vi "Auto_Drive (2).vi"(10 "Target":dbl=40.0 format="%#_13g", 11 "Drive Effort":dbl=0.1) -> ()   [LabVIEW 2016]
uses:
  <vilib>/Rock Robotics/WPI/SafetyOutput/WPI_SafetyOutputConfigMenu.ctl
  Global 2.vi
panel:
  in  "kI":dbl=1.6 format="%#_13g"
  in  "kP":dbl=0.35 format="%#_13g"
  in  "kD":dbl=1.6 format="%#_13g"
  in  "Scaling Factor":dbl=16.0 format="%#_13g"
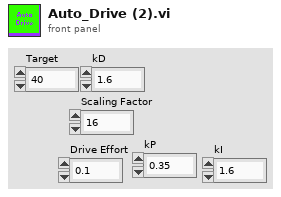
[diagram p1: front panel]
types:
  T1 = typedef "WPI_SafetyOutputConfigMenu.ctl" = enum16{"Enable", "Disable"}
  T2 = typedef "WPI_MotorControlDeviceRef.ctl" = cluster{"DeviceStatus":errorcluster, "Type":T3, "PWM":cluster{"PWM Channel":T4, "DeadBand":T5}, "CAN":cluster{"Device Number":u8, "SetOutput VI Ref":variant, "GetOutput VI Ref":variant, "Enable VI Ref":variant, "Disable VI Ref":variant, "Data":variant}, "Invert":bool}
  T3 = typedef "WPI_MotorControlType.ctl" = enum16{"PWM", "CAN"}
  T4 = typedef "FPGA_DIOPWMChannel.ctl" = enum8{"PWM 0", "PWM 1", "PWM 2", "PWM 3", "PWM 4", "PWM 5", "PWM 6", "PWM 7", "PWM 8", "PWM 9", "PWM MXP 0", "PWM MXP 1", "PWM MXP 2", "PWM MXP 3", "PWM MXP 4", "PWM MXP 5", "PWM MXP 6", "PWM MXP 7", "PWM MXP 8", "PWM MXP 9", "Invalid"}
  T5 = typedef "WPI_PWMDeadband.ctl" = cluster{"Name":string, "maxPositivePwm":i32, "minPositivePwm":i32, "centerPwm":i32, "maxNegativePwm":i32, "minNegativePwm":i32, "angularRange":u16}
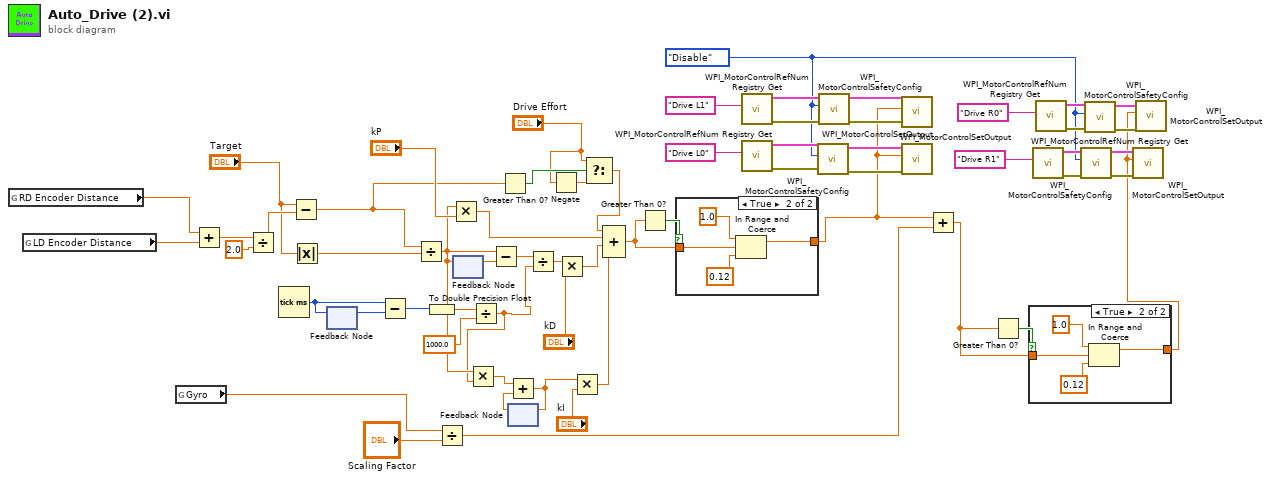
[diagram p0: block diagram]
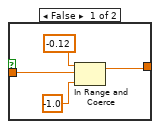
[diagram p2: hidden frame]
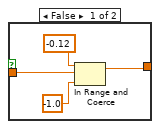
[diagram p3: hidden frame]
diagram:
  w41 = WPI_SafetyOutputConfigMenu."Disable" ("mode")
  n1 = global read "Global 2.vi" "RD Encoder Distance"() -> (w20:dbl)
  n2 = global read "Global 2.vi" "LD Encoder Distance"() -> (w21:dbl)
  n3 = global read "Global 2.vi" "Gyro"() -> (w38:dbl)
  n4 = Add(x=w20, y=w21) -> (x+y=w37:dbl)
  n5 = Divide(x=w37, y=2.0) -> (x/y=w35:dbl)
  n6 = Tick Count (ms)() -> (millisecond timer value=w31:u32)
  n7 = Subtract(x="Target", y=w35) -> (x-y=w15:dbl)
  n8 = Absolute Value(x="Target") -> (abs(x)=w16:dbl)
  n9 = feedback #1() -> (w32:u32)  [unwired: 1 in]
  n10 = feedback-in #1(w31) -> ()
  n11 = Subtract(x=w31, y=w32) -> (x-y=w8:u32)
  n12 = Divide(x=w15, y=w16) -> (x/y=w9:dbl)
  n13 = To Double Precision Float(number=w8) -> (double precision float=w3:dbl)
  n14 = Divide(x=w38, y="Scaling Factor") -> (x/y=w39:dbl)
  n15 = Multiply(x=w9, y="kP") -> (x*y=w27:dbl)
  n16 = feedback #2() -> (w33:dbl)  [unwired: 1 in]
  n17 = feedback-in #2(w9) -> ()
  n18 = Divide(x=w3, y=1000.0) -> (x/y=w1:dbl)
  n19 = Multiply(x=w9, y=w1) -> (x*y=w7:dbl)
  n20 = Subtract(x=w9, y=w33) -> (x-y=w30:dbl)
  n21 = Greater Than 0?(x=w15) -> (x > 0?=w14:bool)
  n22 = feedback #3() -> (w10:dbl)  [unwired: 1 in]
  n23 = Add(x=w7, y=w10) -> (x+y=w6:dbl)
  n24 = feedback-in #3(w6) -> ()
  n25 = Divide(x=w30, y=w1) -> (x/y=w29:dbl)
  n26 = Negate(x="Drive Effort") -> (-x=w13:dbl)
  n27 = Multiply(x=w29, y="kD") -> (x*y=w26:dbl)
  n28 = Multiply(x=w6, y="kI") -> (x*y=w5:dbl)
  n29 = Select(t="Drive Effort", s=w14, f=w13) -> (s? t:f=w11:dbl)
  n30 = Compound Arithmetic op=ADD(w11, w27, w26, w5) -> (w24:dbl)
  n31 = Greater Than 0?(x=w24) -> (x > 0?=w25:bool)
  n32 = case shown="True" w25 {
    tunnel: [w62 w67] -> w23
    tunnel: w24 -> [w63 w66]
    frame False {
      n33 = In Range and Coerce(upper limit=-0.12, x=w63, lower limit=-1.0) -> (coerced(x)=w62:dbl)  [unwired: 1 out]
    }
    frame True {
      n34 = In Range and Coerce(upper limit=1.0, x=w66, lower limit=0.12) -> (coerced(x)=w67:dbl)  [unwired: 1 out]
    }
  }
  n35 = call <vilib>:"WPI_MotorControlRefNum Registry Get.vi"("refnum name"="Drive L1") -> ("error out"=w56:errorcluster, "MotorControlDevRef"=w57:T2)  [unwired: 9 in]
  n36 = call <vilib>:"WPI_MotorControlRefNum Registry Get.vi"("refnum name"="Drive L0") -> ("error out"=w52:errorcluster, "MotorControlDevRef"=w53:T2)  [unwired: 9 in]
  n37 = call <vilib>:"WPI_MotorControlSafetyConfig.vi"("error in (no error)"=w52, "mode"=w41, "MotorControlDevRef"=w53) -> ("error out"=w50:errorcluster, "MotorControlDevRef"=w51:T2)  [unwired: 7 in]
  n38 = call <vilib>:"WPI_MotorControlSafetyConfig.vi"("error in (no error)"=w56, "mode"=w41, "MotorControlDevRef"=w57) -> ("error out"=w54:errorcluster, "MotorControlDevRef"=w55:T2)  [unwired: 7 in]
  n39 = call <vilib>:"WPI_MotorControlSetOutput.vi"("error in (no error)"=w54, "Output"=w23, "MotorControlDevRef"=w55) -> ()  [unwired: 6 in, 3 out]
  n40 = call <vilib>:"WPI_MotorControlSetOutput.vi"("error in (no error)"=w50, "Output"=w23, "MotorControlDevRef"=w51) -> ()  [unwired: 6 in, 3 out]
  n41 = Add(x=w23, y=w39) -> (x+y=w17:dbl)
  n42 = Greater Than 0?(x=w17) -> (x > 0?=w19:bool)
  n43 = case shown="True" w19 {
    tunnel: [w70 w75] -> w18
    tunnel: w17 -> [w71 w74]
    frame False {
      n44 = In Range and Coerce(upper limit=-0.12, x=w71, lower limit=-1.0) -> (coerced(x)=w70:dbl)  [unwired: 1 out]
    }
    frame True {
      n45 = In Range and Coerce(upper limit=1.0, x=w74, lower limit=0.12) -> (coerced(x)=w75:dbl)  [unwired: 1 out]
    }
  }
  n46 = call <vilib>:"WPI_MotorControlRefNum Registry Get.vi"("refnum name"="Drive R1") -> ("error out"=w44:errorcluster, "MotorControlDevRef"=w45:T2)  [unwired: 9 in]
  n47 = call <vilib>:"WPI_MotorControlRefNum Registry Get.vi"("refnum name"="Drive R0") -> ("error out"=w48:errorcluster, "MotorControlDevRef"=w49:T2)  [unwired: 9 in]
  n48 = call <vilib>:"WPI_MotorControlSafetyConfig.vi"("error in (no error)"=w44, "mode"=w41, "MotorControlDevRef"=w45) -> ("error out"=w43:errorcluster, "MotorControlDevRef"=w42:T2)  [unwired: 7 in]
  n49 = call <vilib>:"WPI_MotorControlSafetyConfig.vi"("error in (no error)"=w48, "mode"=w41, "MotorControlDevRef"=w49) -> ("error out"=w47:errorcluster, "MotorControlDevRef"=w46:T2)  [unwired: 7 in]
  n50 = call <vilib>:"WPI_MotorControlSetOutput.vi"("error in (no error)"=w43, "Output"=w18, "MotorControlDevRef"=w42) -> ()  [unwired: 6 in, 3 out]
  n51 = call <vilib>:"WPI_MotorControlSetOutput.vi"("error in (no error)"=w47, "Output"=w18, "MotorControlDevRef"=w46) -> ()  [unwired: 6 in, 3 out]
